vi "Check_IP.vi"(8 "Error In":errorcluster, 11 "Drfiter IP Addresses In":string[][](array[string])) -> (0 "Error Out":errorcluster, 3 "Drfiter IP Addresses Out":string[][](array[string]))   [LabVIEW 2017]
panel:
  out "Terminal Output":string
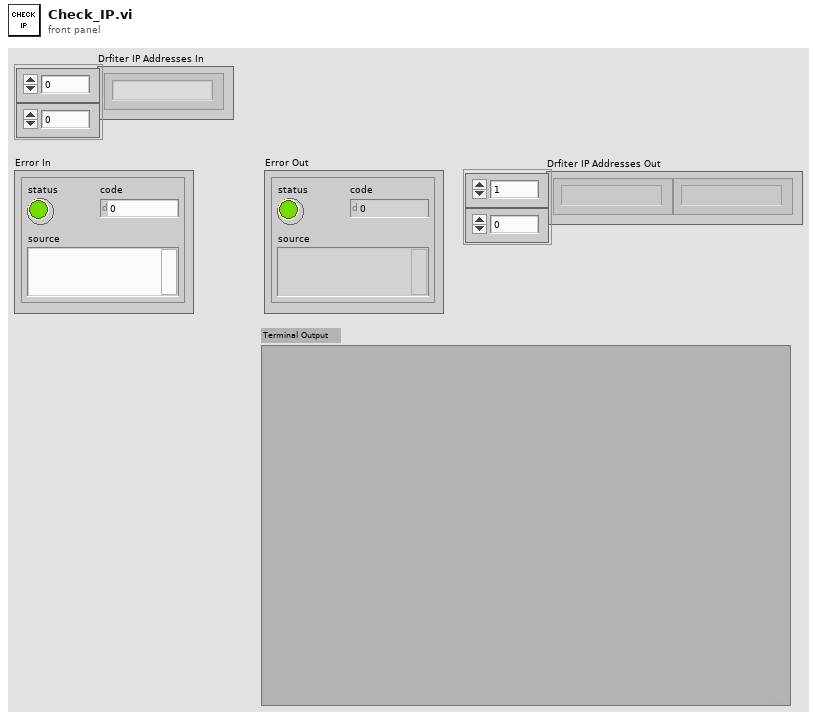
[diagram p1: front panel]
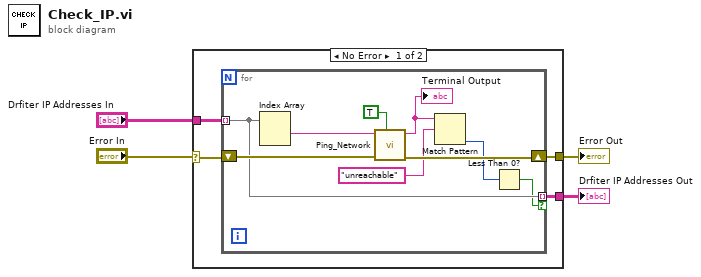
[diagram p0: block diagram]
diagram:
  n1 = case shown="No Error" "Error In" {
    selector: "Error In" -> [w5 w19]
    tunnel: [w8 w19] -> w4
    tunnel: "Drfiter IP Addresses In" -> [w7 w18]
    tunnel: [w6 w18] -> w2
    frame No Error {
      n2 = for {
        tunnel: w7 -> [w10] mode=indexing
        shift-right: [w15] -> w8
        shift-left: w5 -> [w17]
        tunnel: [w10] -> w6 mode=indexing if=w9
        n3 = Index Array(array=w10) -> (element #1=w14:string)  [unwired: 2 in, 1 out]
        n4 = call "Ping_Network.vi"("IP/Default Gateway (T/F)"=TRUE, "Error In"=w17, "Default Gateway/IP"=w14) -> ("Error Out"=w15:errorcluster, "Terminal Output"=w13:string)  [unwired: 7 in]
        "Terminal Output" <- w13
        n5 = Match Pattern(string=w13, regular expression="unreachable") -> (offset past match=w11:i32)  [unwired: 1 in, 3 out]
        n6 = Less Than 0?(x=w11) -> (x < 0?=w9:bool)
      }
    }
    frame Error {
    }
  }
  "Error Out" <- w4
  "Drfiter IP Addresses Out" <- w2
